vi "Handle Error.vi"(8 "error in (no error)":errorcluster, 11 "System Actor in":refnum<class "System Actor.lvclass">) -> (0 "error out":errorcluster, 2 "stop actor?":bool=TRUE, 3 "System Actor out":refnum<class "System Actor.lvclass">)   [LabVIEW 2014, in "Robot Actor Framework.lvlib" / "System Actor.lvlib" / "System Actor.lvclass"]
doc: "(<B>Filename</B>: Actor Framework.lvlib:Actor.lvclass:Handle Error.vi)\n\nDefines how the actor handles an error that occurred while processing a message. By default, this method does nothing except stop the actor."
uses:
  System Actor.lvclass
  <vilib>/ActorFramework/Actor/Actor.lvclass
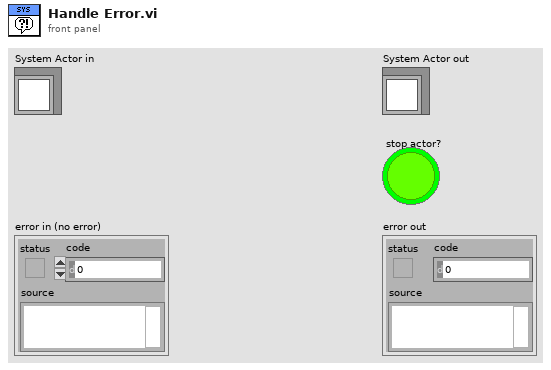
[diagram p1: front panel]
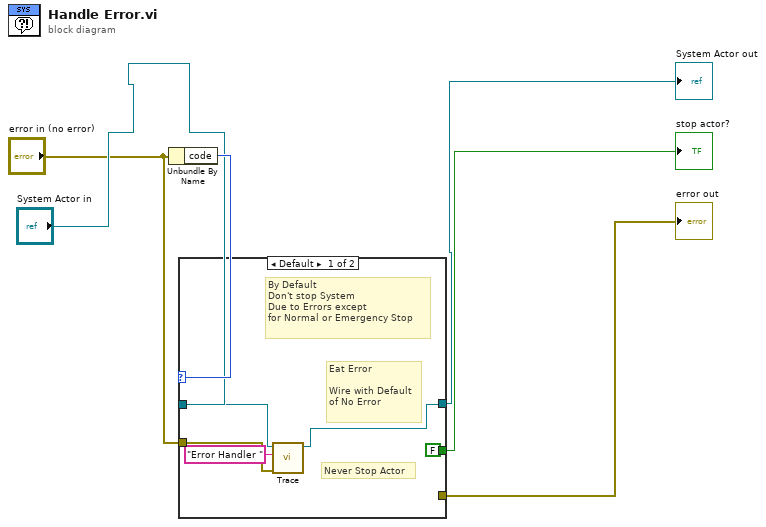
[diagram p0: block diagram]
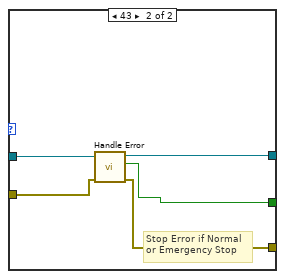
[diagram p2: hidden frame]
diagram:
  n1 = Unbundle By Name("error in (no error)") -> ("code"=w6:i32)
  n2 = case shown="Default" w6 {
    tunnel: [w9 w16] -> w2
    tunnel: [_ w15] -> w1
    tunnel: [FALSE ("stop actor?") w14] -> w5
    tunnel: "System Actor in" -> [w10 w13]
    tunnel: "error in (no error)" -> [w8 w12]
    frame Default {
      # "Never Stop Actor"
      # "Eat Error\n\nWire with Default\nof No Error"
      # "By Default\nDon't stop System\nDue to Errors except\nfor Normal or Emergency Stop"
      n3 = call-dynamic "Trace.vi"("error in (no error)"=w8, "System Action"="Error Handler ", "System Actor in"=w10) -> ("System Actor out"=w9:refnum<class "System Actor.lvclass">)  [unwired: 7 in, 1 out]
    }
    frame 43 {
      # "Stop Error if Normal\nor Emergency Stop"
      n4 = call-parent "Handle Error.vi"("error in (no error)"=w12, "Actor in"=w13) -> ("error out"=w15:errorcluster, "stop actor?"=w14:bool, "Actor out"=w16:refnum<class "System Actor.lvclass">)  [unwired: 7 in]
    }
  }
  "System Actor out" <- w2
  "error out" <- w1
  "stop actor?" <- w5
